vi "pixel_select_handler.vi"(3 "Wavelength":dbl, 5 "Scrollbar V":i32, 6 "Pixels":i32[](array[numeric]), 7 "Pixel":i32, 8 "Wavelengths":dbl[](array[numeric]), 9 "Voltages":dbl[](array[numeric]), 10 "Zeroes (idx)":cluster{"Splice indices":i32[]}[](array[cluster]), 11 "Curr idx":u32) -> (2 "New idx":u32)   [LabVIEW 2019]
uses:
  REFS.vi
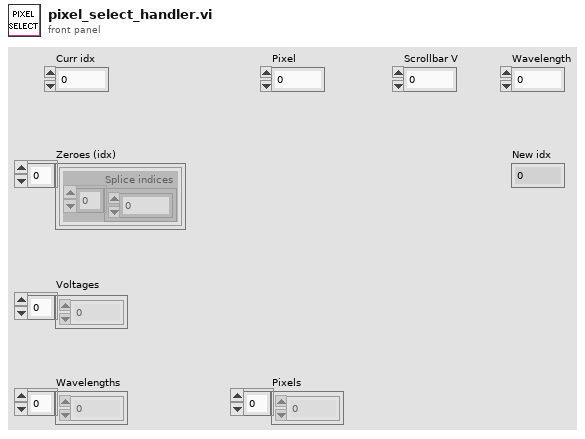
[diagram p1: front panel]
types:
  T1 = cluster{string, i32, i32, i32, bool, bool, i32, i32, i32, cluster{"Numeric":dbl, dbl}, i32, i32, i32[], bool, i32, cluster{dbl, dbl}}
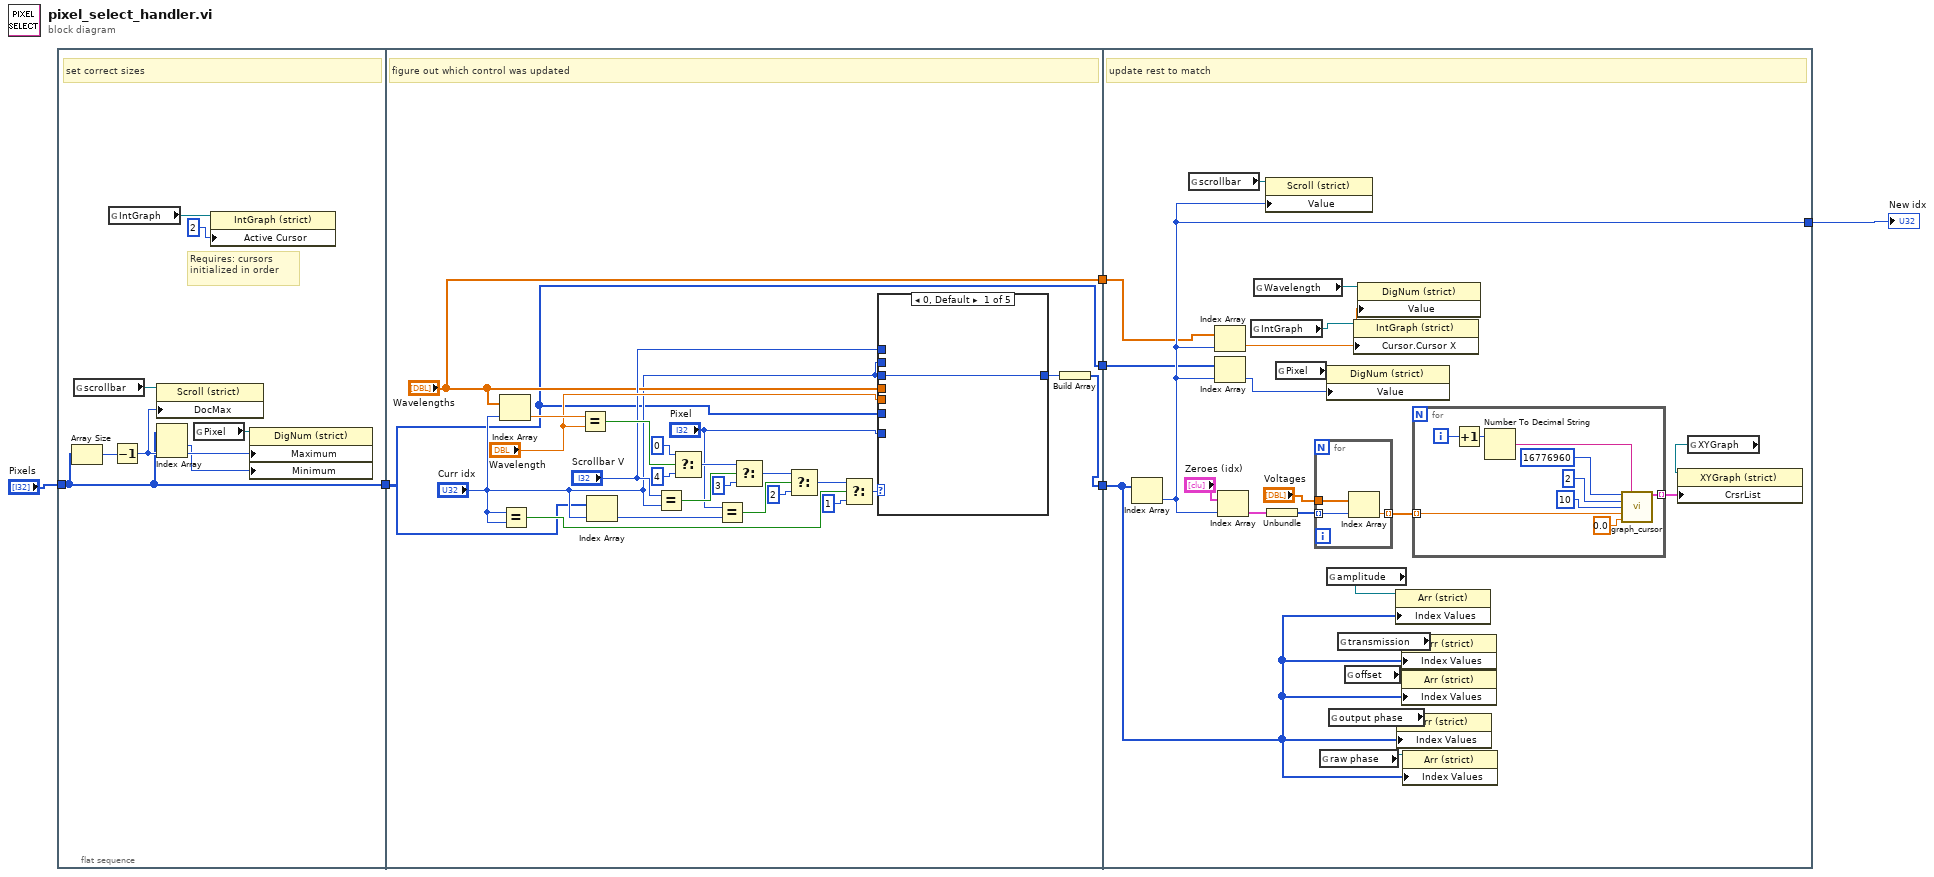
[diagram p0: block diagram]
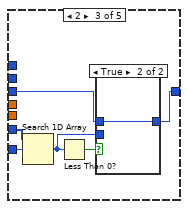
[diagram p3: hidden frame]
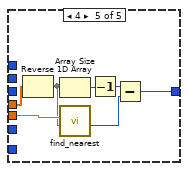
[diagram p6: hidden frame]
diagram:
  n1 = flat-sequence {
    tunnel: [w7] -> w4
    tunnel: "Pixels" -> [w7]
    tunnel: [w26] -> w6
    tunnel: w4 -> [w16]
    tunnel: ["Wavelengths"] -> w3
    tunnel: [w16] -> w1
    tunnel: [w76] -> w5
    tunnel: w6 -> [w77]
    tunnel: w3 -> [w60]
    tunnel: w1 -> [w59]
    frame #0 {
      # "Requires: cursors initialized in order"
      # "set correct sizes"
      n2 = Array Size(array=w7) -> (size(s)=w14:i32)
      n3 = global read "REFS.vi" "scrollbar"() -> (w9:refnum<vi>)
      n4 = global read "REFS.vi" "IntGraph"() -> (w10:refnum<vi>)
      n5 = Decrement(x=w14) -> (x-1=w11:i32)
      n6 = property on="Property Node" class="Scroll (strict)"(reference=w9, "DocMax"=w11) -> ()  [unwired: 1 in, 2 out]
      n7 = Index Array(array=w7, index #2=w11) -> (element #1=w12:i32, element #2=w13:i32)  [unwired: 1 in]
      n8 = global read "REFS.vi" "Pixel"() -> (w8:refnum<vi>)
      n9 = property on="Property Node" class="IntGraph (strict)"(reference=w10, "Active Cursor"=u32 2) -> ()  [unwired: 1 in, 2 out]
      n10 = property on="Property Node" class="DigNum (strict)"(reference=w8, "Maximum"=w13, "Minimum"=w12) -> ()  [unwired: 1 in, 2 out]
    }
    frame #1 {
      # "figure out which control was updated"
      n11 = Index Array(array="Wavelengths", index="Curr idx") -> (element=w23:dbl)
      n12 = Equal?(x="Curr idx", y="Curr idx") -> (x = y?=w38:bool)
      n13 = Equal?(x=w23, y="Wavelength") -> (x = y?=w32:bool)
      n14 = Index Array(array=w16, index="Curr idx") -> (element=w22:i32)
      n15 = Equal?(x="Scrollbar V", y="Curr idx") -> (x = y?=w24:bool)
      n16 = Select(t=0, s=w32, f=4) -> (s? t:f=w33:i32)
      n17 = Equal?(x="Pixel", y=w22) -> (x = y?=w25:bool)
      n18 = Select(t=w33, s=w24, f=3) -> (s? t:f=w34:i32)
      n19 = Select(t=w34, s=w25, f=2) -> (s? t:f=w35:i32)
      n20 = Select(t=w35, s=w38, f=1) -> (s? t:f=w37:i32)
      n21 = case shown="0, Default" w37 {
        tunnel: "Wavelength" -> [_ _ _ _ w56]
        tunnel: "Curr idx" -> [w39 _ w41 _ _]
        tunnel: [w39 w40 w42 w49 w50] -> w27
        tunnel: "Curr idx" -> [_ w40 _ _ _]
        tunnel: "Pixel" -> [_ _ w46 _ _]
        tunnel: "Scrollbar V" -> [_ _ _ w49 _]
        tunnel: "Wavelengths" -> [_ _ _ _ w55]
        tunnel: w16 -> [_ _ w45 _ _]
        frame 0, Default {
        }
        frame 1 {
        }
        frame 2 {
          n22 = Search 1D Array(1D array=w45, element=w46) -> (index of element=w43:i32)  [unwired: 1 in]
          n23 = Less Than 0?(x=w43) -> (x < 0?=w44:bool)
          n24 = case shown="True" w44 {
            tunnel: w43 -> [w47 _]
            tunnel: [w47 w48] -> w42
            tunnel: w41 -> [_ w48]
            frame False {
            }
            frame True {
            }
          }
        }
        frame 3 {
        }
        frame 4 {
          n25 = Reverse 1D Array(array=w55) -> (reversed array=w53:dbl[])
          n26 = Array Size(array=w53) -> (size(s)=w54:i32)
          n27 = call "find_nearest.vi"("Sorted Array (<)"=w53, "Key"=w56) -> ("Nearest index"=w51:i32)  [unwired: 6 in, 3 out]
          n28 = Decrement(x=w54) -> (x-1=w52:i32)
          n29 = Subtract(x=w52, y=w51) -> (x-y=w50:i32)
        }
      }
      n30 = Build Array(w27) -> (w26:u32[])
    }
    frame #2 {
      # "update rest to match"
      n31 = Index Array(array=w77) -> (element=w76:u32)  [unwired: 1 in]
      n32 = global read "REFS.vi" "scrollbar"() -> (w64:refnum<vi>)
      n33 = Index Array(array=w60, index=w76) -> (element=w74:dbl)
      n34 = Index Array(array=w59, index=w76) -> (element=w78:i32)
      n35 = Index Array(array="Zeroes (idx)", index=w76) -> (element=w72:cluster{"Splice indices":i32[]})
      n36 = global read "REFS.vi" "IntGraph"() -> (w65:refnum<vi>)
      n37 = global read "REFS.vi" "Wavelength"() -> (w62:refnum<vi>)
      n38 = property class="Scroll (strict)"(reference=w64, "Value"=w76) -> ()  [unwired: 1 in, 2 out]
      n39 = Unbundle(w72) -> ("Splice indices"=w71:i32[])
      n40 = global read "REFS.vi" "Pixel"() -> (w63:refnum<vi>)
      n41 = for {
        tunnel: w71 -> [w81] mode=indexing
        tunnel: "Voltages" -> [w80]
        tunnel: [w79] -> w73 mode=indexing
        n42 = Index Array(array=w80, index=w81) -> (element=w79:dbl)
      }
      n43 = global read "REFS.vi" "raw phase"() -> (w66:refnum<vi>)
      n44 = property class="DigNum (strict)"(reference=w63, "Value"=w78) -> ()  [unwired: 1 in, 2 out]
      n45 = global read "REFS.vi" "amplitude"() -> (w70:refnum<vi>)
      n46 = global read "REFS.vi" "output phase"() -> (w67:refnum<vi>)
      n47 = global read "REFS.vi" "transmission"() -> (w68:refnum<vi>)
      n48 = global read "REFS.vi" "offset"() -> (w69:refnum<vi>)
      n49 = property on="Property Node" class="IntGraph (strict)"(reference=w65, "Cursor.Cursor X"=w74) -> ()  [unwired: 1 in, 2 out]
      n50 = property class="DigNum (strict)"(reference=w62, "Value"=w74) -> ()  [unwired: 1 in, 2 out]
      n51 = property on="Property Node" class="Arr (strict)"(reference=w70, "Index Values"=w77) -> ()  [unwired: 1 in, 2 out]
      n52 = property on="Property Node" class="Arr (strict)"(reference=w67, "Index Values"=w77) -> ()  [unwired: 1 in, 2 out]
      n53 = property on="Property Node" class="Arr (strict)"(reference=w68, "Index Values"=w77) -> ()  [unwired: 1 in, 2 out]
      n54 = property on="Property Node" class="Arr (strict)"(reference=w69, "Index Values"=w77) -> ()  [unwired: 1 in, 2 out]
      n55 = property on="Property Node" class="Arr (strict)"(reference=w66, "Index Values"=w77) -> ()  [unwired: 1 in, 2 out]
      n56 = for {
        tunnel: [w89] -> w75 mode=indexing
        tunnel: w73 -> [w88] mode=indexing
        i -> [w82]
        n57 = Increment(x=w82) -> (x+1=w83:i32)
        n58 = Number To Decimal String(number=w83) -> (decimal integer string=w84:string)  [unwired: 1 in]
        n59 = call "graph_cursor.vi"("Colour"=16776960, "Name"=w84, "Style"=2, "Point style"=10, "X"=w88, "Y"=0.0) -> ("Cursor Cluster"=w89:T1)  [unwired: 9 in]
      }
      n60 = global read "REFS.vi" "XYGraph"() -> (w61:refnum<vi>)
      n61 = property on="Property Node" class="XYGraph (strict)"(reference=w61, "CrsrList"=w75) -> ()  [unwired: 1 in, 2 out]
    }
  }
  "New idx" <- w5
